vi "Test.vi"() -> ()   [LabVIEW 2025]
panel:
  out "Voltaje":dbl
  in  "DAC":u8(knob) scale=0.0..255.0
  out "unsigned byte array":u8[](array[numeric])
  out "Analog read":u16
  in  "Estado":bool
  out "Valor":bool
  in  "Pin PWM":u8=4 min=4 max=40
  in  "DC":u8(slide) scale=0.0..255.0
  in  "Color Box 2":u32(colorbox)
  in  "Color Box":u32(colorbox)
  in  "No. NeoPixel":u8=1 max=2
  in  "PIN AO":u8=4 min=4 max=40
  in  "PIN AI":u8=4 min=4 max=40
  in  "PIN DOUT":u8=4 min=4 max=40
  in  "PIN DIN":u8=4 min=4 max=40
  in  "stop":bool
  out "error out":errorcluster
  in  "PWM":bool
  in  "NEOs":bool
  in  "NEO":bool
  in  "AOUT":bool
  in  "AIN":bool
  in  "DOUT":bool
  in  "DIN":bool
  in  "VISA resource name":refnum<visa-resource-name>
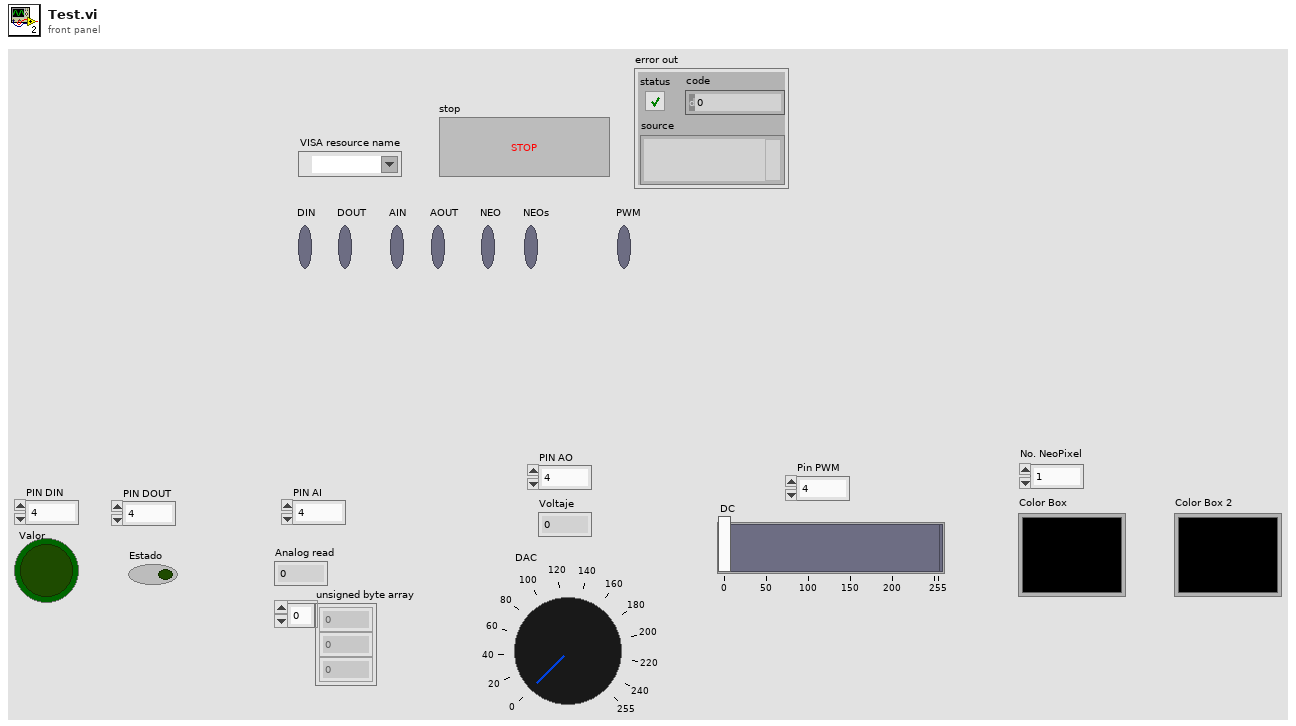
[diagram p1: front panel]
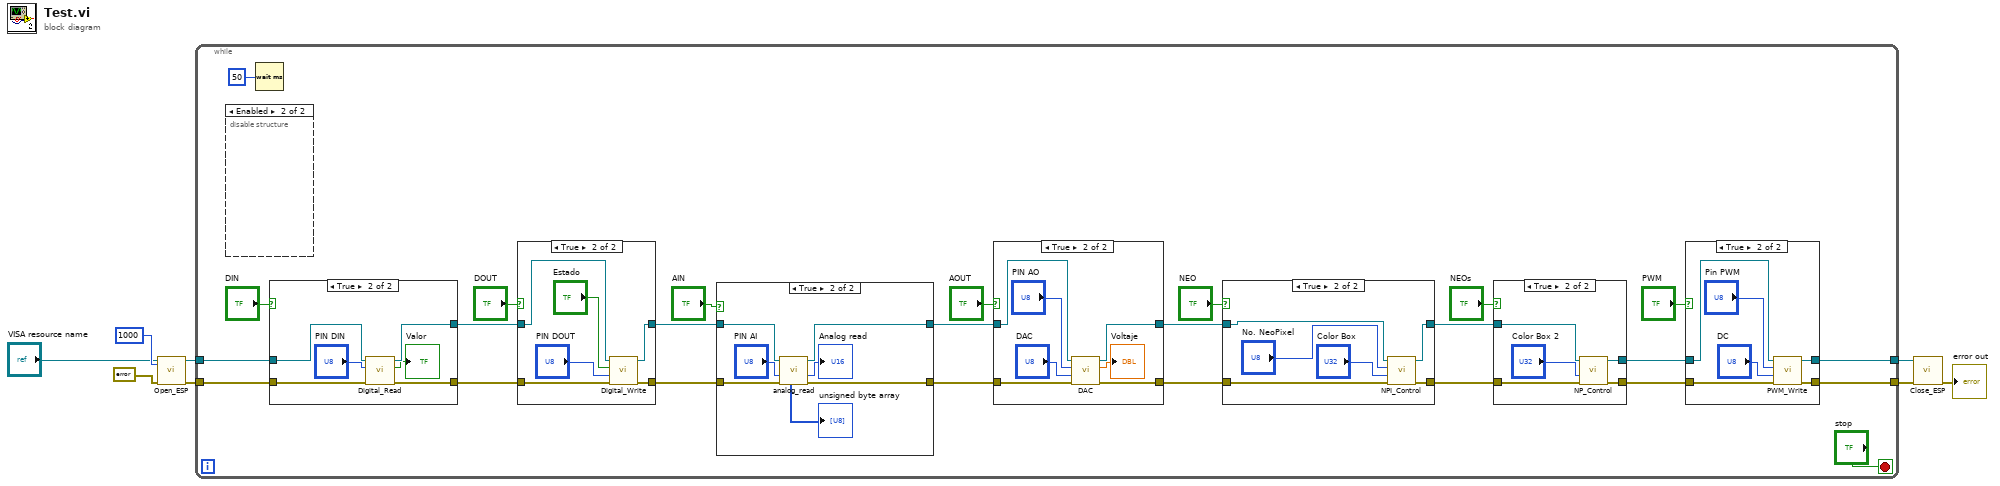
[diagram p0: block diagram]
diagram:
  n1 = call "Open_ESP.vi"("timeout (10sec)"=u32 1000, "error in (no error)"=errorcluster {"status"=FALSE, "code"=0, "source"=""}, "VISA resource name"="VISA resource name") -> ("error out"=w1:errorcluster, "VISA resource name out"=w4:refnum<visa-resource-name>)  [unwired: 7 in]
  n2 = while {
    tunnel: w4 -> [w26]
    tunnel: [w19] -> w3
    tunnel: [w18] -> w2
    tunnel: w1 -> [w11]
    stop <- "stop" stop-if-true
    n3 = disable-structure shown="Enabled" {
      frame Disabled {
      }
      frame Enabled {
      }
    }
    n4 = Wait (ms)(milliseconds to wait=u32 50) -> ()  [unwired: 1 out]
    n5 = case shown="True" "DIN" {
      tunnel: w26 -> [w84 w90]
      tunnel: [w84 w89] -> w25
      tunnel: [w83 w88] -> w12
      tunnel: w11 -> [w83 w87]
      frame False {
      }
      frame True {
        n6 = call "Digital_Read.vi"("error in (no error)"=w87, "Pin"="PIN DIN", "VISA resource name"=w90) -> ("error out"=w88:errorcluster, "Valor"=→"Valor":bool, "VISA resource name out"=w89:refnum<visa-resource-name>)  [unwired: 6 in]
      }
    }
    n7 = case shown="True" "DOUT" {
      tunnel: w25 -> [w76 w82]
      tunnel: [w76 w81] -> w24
      tunnel: [w75 w80] -> w13
      tunnel: w12 -> [w75 w79]
      frame False {
      }
      frame True {
        n8 = call "Digital_Write.vi"("error in (no error)"=w79, "Pin"="PIN DOUT", "Estado"="Estado", "VISA resource name"=w82) -> ("error out"=w80:errorcluster, "VISA resource name out"=w81:refnum<visa-resource-name>)  [unwired: 6 in]
      }
    }
    n9 = case shown="True" "AIN" {
      tunnel: w24 -> [w67 w74]
      tunnel: [w67 w73] -> w23
      tunnel: [w66 w72] -> w14
      tunnel: w13 -> [w66 w71]
      frame False {
      }
      frame True {
        n10 = call "analog_read.vi"("error in (no error)"=w71, "Pin"="PIN AI", "VISA resource name"=w74) -> ("error out"=w72:errorcluster, "Analog read"=→"Analog read":u16, "VISA resource name out"=w73:refnum<visa-resource-name>, "unsigned byte array"=→"unsigned byte array":u8[])  [unwired: 5 in]
      }
    }
    n11 = case shown="True" "AOUT" {
      tunnel: w23 -> [w57 w65]
      tunnel: [w57 w64] -> w22
      tunnel: [w58 w63] -> w15
      tunnel: w14 -> [w58 w62]
      frame False {
      }
      frame True {
        n12 = call "DAC.vi"("error in (no error)"=w62, "DAC"="DAC", "Pin"="PIN AO", "VISA resource name"=w65) -> ("error out"=w63:errorcluster, "Voltaje"=→"Voltaje":dbl, "VISA resource name out"=w64:refnum<visa-resource-name>)  [unwired: 5 in]
      }
    }
    n13 = case shown="True" "NEO" {
      tunnel: w22 -> [w50 w56]
      tunnel: [w50 w55] -> w21
      tunnel: [w49 w54] -> w16
      tunnel: w15 -> [w49 w53]
      frame False {
      }
      frame True {
        n14 = call "NPI_Control.vi"("error in (no error)"=w53, "Color Box"="Color Box", "No. NeoPixel"="No. NeoPixel", "VISA resource name"=w56) -> ("error out"=w54:errorcluster, "VISA resource name out"=w55:refnum<visa-resource-name>)  [unwired: 6 in]
      }
    }
    n15 = case shown="True" "NEOs" {
      tunnel: w21 -> [w42 w48]
      tunnel: [w42 w47] -> w20
      tunnel: [w43 w46] -> w17
      tunnel: w16 -> [w43 w45]
      frame False {
      }
      frame True {
        n16 = call "NP_Control.vi"("error in (no error)"=w45, "Color Box"="Color Box 2", "VISA resource name"=w48) -> ("error out"=w46:errorcluster, "VISA resource name out"=w47:refnum<visa-resource-name>)  [unwired: 7 in]
      }
    }
    n17 = case shown="True" "PWM" {
      tunnel: w20 -> [w35 w41]
      tunnel: [w35 w40] -> w19
      tunnel: [w34 w39] -> w18
      tunnel: w17 -> [w34 w38]
      frame False {
      }
      frame True {
        n18 = call "PWM_Write.vi"("error in (no error)"=w38, "DC"="DC", "Pin"="Pin PWM", "VISA resource name"=w41) -> ("error out"=w39:errorcluster, "VISA resource name out"=w40:refnum<visa-resource-name>)  [unwired: 6 in]
      }
    }
  }
  n19 = call "Close_ESP.vi"("error in (no error)"=w2, "VISA resource name"=w3) -> ("error out"=→"error out":errorcluster)  [unwired: 9 in]
